vi "Pose3d_New_Default.vi"() -> (3 "outPose3d":T1={"Translation3d"={"X"=0.0, "Y"=0.0, "Z"=0.0}, "Rotation3d"={"Q_quaternion"={"R"=1.0, "V"=[0.0, 0.0, 0.0]}}} {"Translation3d"."Z" format="%14.3f"; "Translation3d"."Y" format="%14.3f"; "Translation3d"."X" format="%14.3f"})   [LabVIEW 2019, in "Trajectory_Library.lvlib"]
doc: "Constructs a pose with the specified translation and rotation.\n\nParameters:\n - translation - The translational component of the pose.\n - rotation - The rotational component of the pose.\n\nReturn:\n - POSE - Pose data structure"
uses:
  Trajectory_Library.lvlib
  TRANSLATION3D.ctl
  QUATERNION.ctl
  ROTATION3D.ctl
  POSE3D.ctl
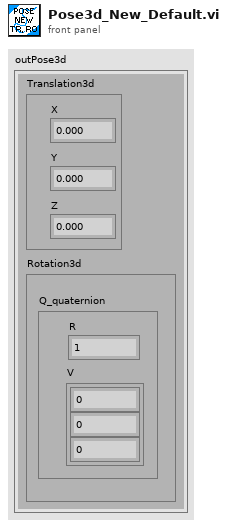
[diagram p1: front panel]
types:
  T1 = typedef "Trajectory_Library.lvlib/POSE3D.ctl" = cluster{"Translation3d":T2, "Rotation3d":T3}
  T2 = typedef "Trajectory_Library.lvlib/TRANSLATION3D.ctl" = cluster{"X":dbl, "Y":dbl, "Z":dbl}
  T3 = typedef "Trajectory_Library.lvlib/ROTATION3D.ctl" = cluster{"Q_quaternion":T4}
  T4 = typedef "Trajectory_Library.lvlib/QUATERNION.ctl" = cluster{"R":dbl, "V":dbl[]}
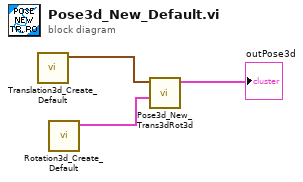
[diagram p0: block diagram]
diagram:
  n1 = call "Translation3d_Create_Default.vi"() -> ("TRANSLATION3D"=w3:T2)  [unwired: 11 in]
  n2 = call "Rotation3d_Create_Default.vi"() -> ("ROTATION3D"=w2:T3)  [unwired: 11 in]
  n3 = call "Pose3d_New_Trans3dRot3d.vi"("Rotation3d"=w2, "Translation3d"=w3) -> ("outPose3d"=→"outPose3d":T1)  [unwired: 9 in]
